vi "MirrorChannelTest.vi"() -> ()   [LabVIEW 2014]
uses:
  TypeDef/GalvoInput.ctl
panel:
  in  "stop":bool
  in  "Scan":bool
  out "Waveform Graph":waveform(dbl)[](graph)=[{"t0"=timestamp(0 s since 1904-01-01), "dt"=0.001, "Y"=[]}]
  out "Sample Rate":dbl=1000.0 format="%0.2f"
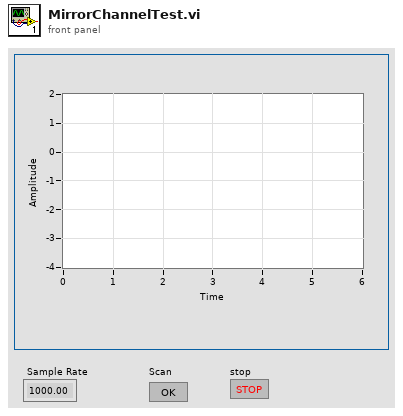
[diagram p1: front panel]
types:
  T1 = typedef "GalvoInput.ctl" = cluster{"Sample Rate":dbl, "Sample Clock Source":tag, "Max Voltage":dbl, "Min Voltage":dbl, "Physical Channel(s)":tag}
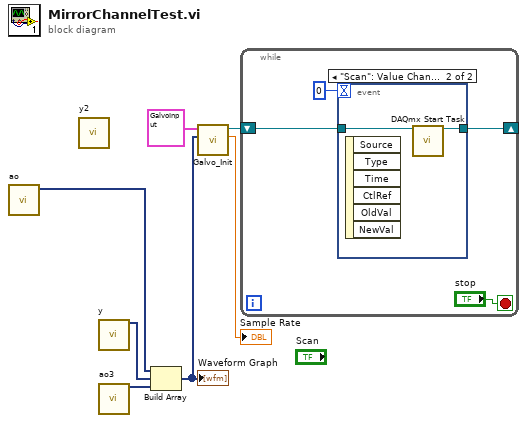
[diagram p0: block diagram]
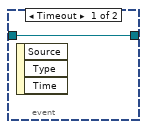
[diagram p2: hidden frame]
diagram:
  n1 = call "ao"() -> ("Signal"=w1:dynamicdata)  [unwired: 9 in, 2 out]
  n2 = call "y2"() -> ()  [unwired: 14 in, 2 out]
  n3 = call "y"() -> ("Sine"=w6:dynamicdata)  [unwired: 14 in, 1 out]
  n4 = call "ao3"() -> ("Sine"=w5:dynamicdata)  [unwired: 14 in, 1 out]
  n5 = Build Array(w1, w6, w5) -> (w3:dynamicdata[])
  "Waveform Graph" <- w3
  n6 = call "Galvo_Init.vi"("Signal array"=w3, "Galvo_Input"=T1 {"Sample Rate"=1000.0, "Sample Clock Source"="OnboardClock", "Max Voltage"=10.0, "Min Voltage"=-10.0, "Physical Channel(s)"="Dev1/ao0,Dev1/ao1,Dev1/ao3"} ("Galvo1_1")) -> ("Actual Sample Rate"=→"Sample Rate":dbl, "task out"=w2:refnum<k21>)  [unwired: 7 in, 1 out]
  n7 = while {
    shift-right: [w8] -> _
    shift-left: w2 -> [w9]
    stop <- "stop" stop-if-true
    n8 = event shown="[1] \"Scan\": Value Change" {
      selector: _ -> [_ _]
      dyn-events: _ -> [_ _]
      timeout: 0 -> [_ _]
      tunnel: w9 -> [w12 w14]
      tunnel: [w12 w13] -> w8
      event Timeout {
        n9 = event-data() -> ()  [unwired: 1 in, 3 out]
      }
      event "Scan": Value Change {
        n10 = event-data() -> ()  [unwired: 1 in, 6 out]
        n11 = call <vilib>:"DAQmx Start Task.vi"("task/channels in"=w14) -> ("task out"=w13:refnum<k21>)  [unwired: 13 in, 1 out]
      }
    }
  }
